vi "array to filter array.vi"(4 "keep elements?":bool[](array[boolean])) -> (1 "insertion list":i32[](array[numeric]))   [LabVIEW 2012]
doc: "This VI helps build a filtered array (which should really be a built-in LabVIEW function). See the front panel for the example code showing how to use this VI!!!\n\nJWD FEB 2006\n\nMinor performance tweaks since I use this heavily. RBC APR 2006"
panel:
  # "disable indexing!"
  # "This shows how to use this VI."
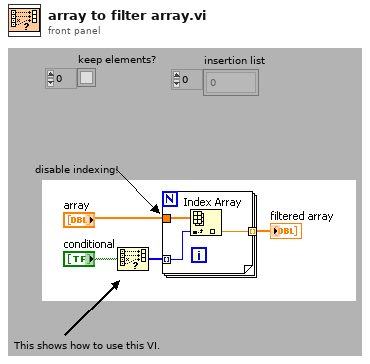
[diagram p1: front panel]
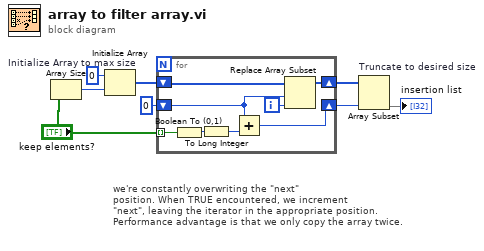
[diagram p0: block diagram]
diagram:
  # "we're constantly overwriting the \"next\"\nposition. When TRUE encountered, we increment\n\"next\", leaving the iterator in the appropriate position.\nPerformance advantage is that we only copy the array twice."
  n1 = Array Size(array="keep elements?") -> (size(s)=w6:i32)
  n2 = Initialize Array "Initialize Array to max size"(0, w6) -> (w8:i32[])
  n3 = for {
    tunnel: "keep elements?" -> [w14] mode=indexing
    shift-right: [w15] -> w4
    shift-left: w8 -> [w16]
    shift-right: [w10] -> w3
    shift-left: 0 -> [w9]
    i -> [w11]
    n4 = Boolean To (0,1)(Boolean=w14) -> (0, 1=w13:i16)
    n5 = To Long Integer(number=w13) -> (32bit integer=w12:i32)
    n6 = Add(x=w9, y=w12) -> (x+y=w10:i32)
    n7 = Replace Array Subset(array=w16, new element=w11, index=w9) -> (w15:i32[])
  }
  n8 = Array Subset "Truncate to desired size"(array=w4, length=w3) -> (→"insertion list":i32[])  [unwired: 1 in]
